vi "FPGA-SRAM-Top-Level.vi"() -> ()   [LabVIEW 2015]
uses:
  Typedefs/RadioData to SRAM states.ctl
  Typedefs/read from SRAM states.ctl
  <vilib>/Platform/TimedLoop/XDataNode/timing_clust.ctl
  <vilib>/Platform/TimedLoop/XDataNode/nitl_modes.ctl
  <vilib>/Platform/TimedLoop/XDataNode/wakeup.ctl
  <vilib>/rvi/Emulation/niFpgaSctlEmulationGetInTimedLoop.vi
  <vilib>/rvi/Emulation/niFpgaEmulationReportErrorSimple.vi
  <vilib>/rvi/Emulation/niFpgaGetClockAttributes.vi
  <vilib>/rvi/Emulation/niFpgaCriticalErrorInLSC.vi
  <vilib>/rvi/interface/RandomDataEmulation/niFpgaRandomDataHandleErrors.vi
  <vilib>/rvi/Emulation/niFpgaEmulationIsFPGAContextNoSignature.vi
  <vilib>/rvi/errors/niFpgaSetErrorForExecOnDevCompSimple.vi
  <vilib>/rvi/eio/common/nirviEmuReportErrorAndStop.vi
  <vilib>/rvi/DataTransferAndStorage/Container/Common/niFpgaContainerGetUniqueNameForEmu.vi
  <vilib>/rvi/FIFO/Fifo_Resource/nirvififoEmulationSetSize.vi
  <vilib>/rvi/FIFO/Fifo_Resource/nirviFifoEmulationQueueMgr.vi
  <instcachedir>/0/nirviFifoEmulationQueueMgr_E5CAEC123FF24DC58D834DCA3CDAA9B5.lvgen/nirviFifoEmulationQueueMgr_E5CAEC123FF24DC58D834DCA3CDAA9B5_001.vi
  <vilib>/rvi/FIFO/Fifo_Resource/nirvififoEmulationDetermineInputValidOut.vi
  <vilib>/rvi/FIFO/Fifo_Resource/nirvififoEmulationCreateLock.vi
  <vilib>/rvi/Emulation/niFpgaProcessEmulError.vi
  <vilib>/rvi/FIFO/Fifo_Resource/nirvififoEmulationObtainLock.vi
  <vilib>/rvi/FIFO/Fifo_Resource/nirvififoEmulationReleaseLock.vi
  <vilib>/rvi/occurrence/nirviWaitOnOccurrenceBase.vi
  <vilib>/rvi/errors/nirviReportUnexpectedCaseInternalError.vi
  <vilib>/rvi/errors/nirviReportUnexpectedCaseInternalError (U32).vi
  <vilib>/rvi/DataTransferAndStorage/Container/Common/niFpgaContainerSetEmuInfo.vi
  <vilib>/Utility/error.llb/Clear Errors.vi
  <vilib>/rvi/Memory/Memory_Emulation/nirvimemoryFastEmulation.vi
  <vilib>/rvi/Memory/Memory_Emulation/nirvimemoryEmulation.vi
  <vilib>/Platform/TimedLoop/XDataNode/XDataNode.xnode
  <vilib>/rvi/DataTransferAndStorage/Container/XNode/niFpgaContainer.xnode
  <vilib>/rvi/interface/RandomDataEmulation/nirviRandomDataFpgaReadWriteTemplate.vi
  <vilib>/rvi/FIFO/Fifo_Resource/nirvififoEmulationWrite.vi
  <vilib>/rvi/LocalResourceManager/LocalResourceManager.xnode
  <vilib>/rvi/FIFO/Fifo_Resource/nirvififoEmulationGetNumberOfElementsToRead.vi
  <vilib>/rvi/FIFO/Fifo_Resource/nirvififoEmulationRead.vi
  <vilib>/Platform/TimedLoop/XDataNode/XDNodeRunTimeDep.lvlib
  Shared/FPGA_shared.lvlib
  Typedefs/SRAM-typedefs.lvlib
  <instrlib>/_niInstr/Basic Elements/v1/FPGA/niInstr Basic Elements v1 FPGA.lvlib
panel:
  out "Target to Host Count":u32
  out "TH Timeout?":bool
  out "from SRAM timeout?":bool
  in  "Reset Read SRAM":bool=TRUE
  out "Radio Data Count to SRAM":u32
  out "Memory Write Address (indicator)":u32
  in  "Reset Write to SRAM":bool=TRUE
  out "HT Timeout?":bool
  out "Host to Target Count":u32
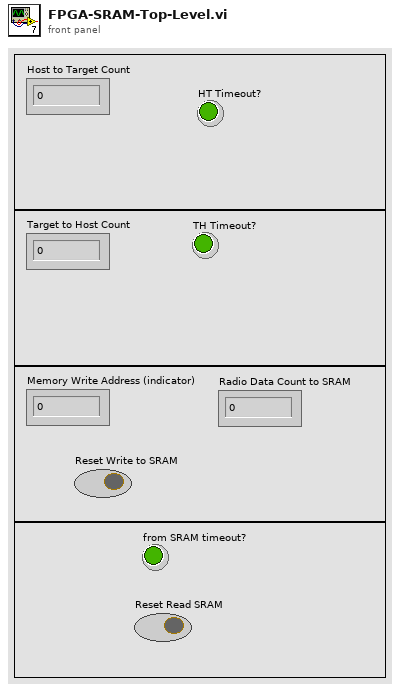
[diagram p1: front panel]
types:
  T1 = typedef "SRAM-typedefs.lvlib/read from SRAM states.ctl" = enum16{"idle", "read"}
  T2 = typedef "SRAM-typedefs.lvlib/RadioData to SRAM states.ctl" = enum16{"idle", "write", "reset"}
  T3 = typedef "XDNodeRunTimeDep.lvlib/timing_clust.ctl" = cluster{"Expected End [f-1]":u64, "Actual End [f-1]":u64, "Finished Late? [f-1]":bool, "Expected End [i-1]":u64, "Actual End [i-1]":u64, "Finished Late? [i-1]":bool, "Expected Start [i]":u64, "Actual Start [i]":u64, "Expected Start [f]":u64, "Actual Start [f]":u64, "Source Name":string, "Structure Name":string, "Period":i64, "Deadline":i64, "Offset":i64, "Start":i64, "Priority":i32, "Timeout":i32, "Mode":T4, "Wakeup Reason":T5, "Error":errorcluster, "Source Type":string, "Secondary Source Type":string, "Global End Time":u64, "Global Start Time":u64, "Frame Duration":u64, "Iteration Duration":u64, "Assigned CPU":i32, "I/O Scan Engine Mode":u32}
  T4 = typedef "XDNodeRunTimeDep.lvlib/nitl_modes.ctl" = enum32{"No Change", "Process missed periods, maintain original phase", "Discard missed periods, maintain original phase", "Process missed periods, ignore original phase", "Discard missed periods, ignore original phase"}
  T5 = typedef "XDNodeRunTimeDep.lvlib/wakeup.ctl" = enum32{"Normal", "Aborted", "Asynchronous wakeup", "Timing source error", "Timed loop error", "Timeout"}
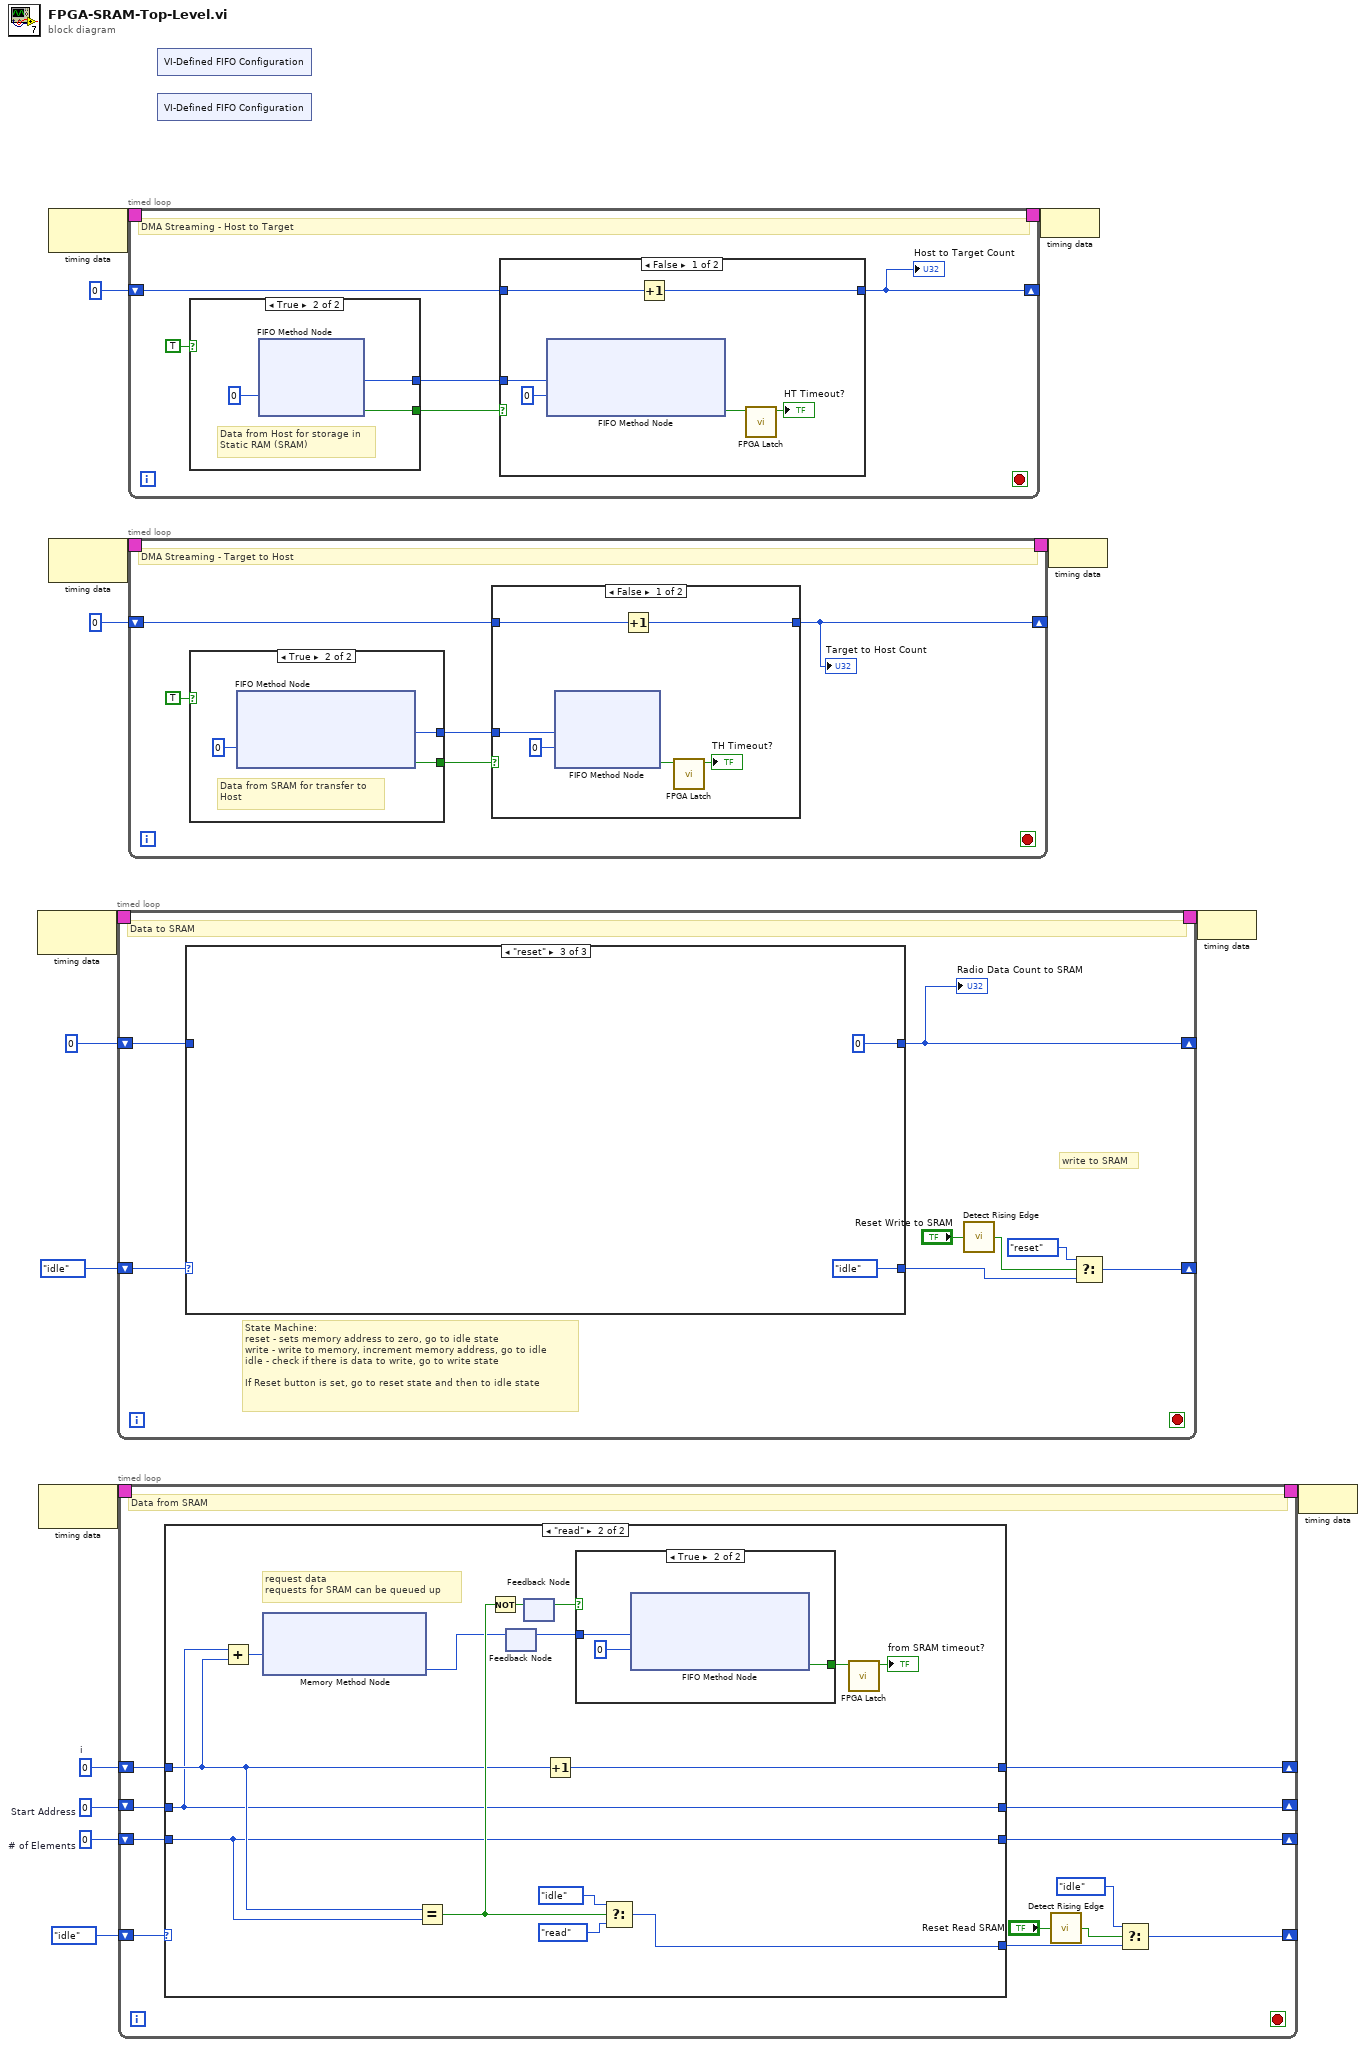
[diagram p0: block diagram]
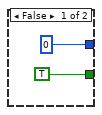
[diagram p2: hidden frame]
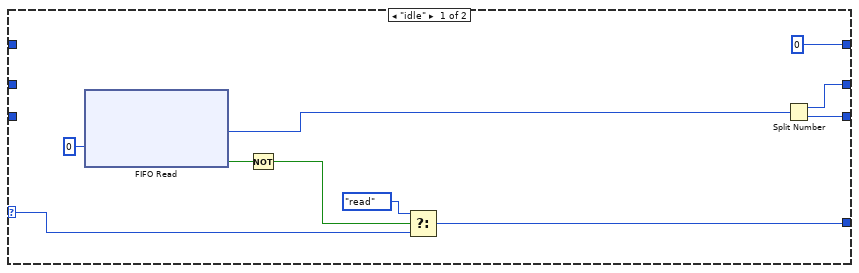
[diagram p4: hidden frame]
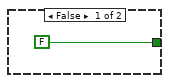
[diagram p5: hidden frame]
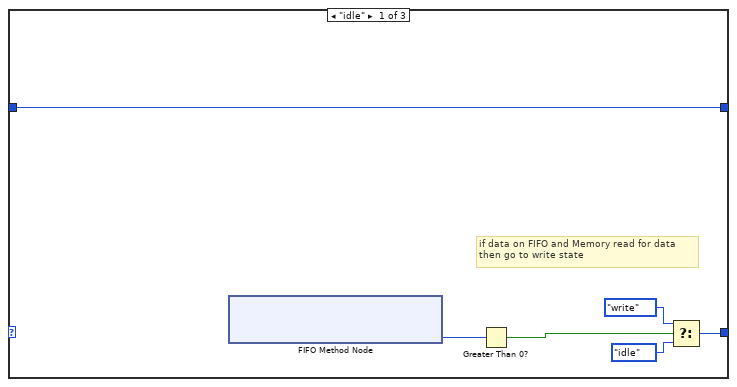
[diagram p6: hidden frame]
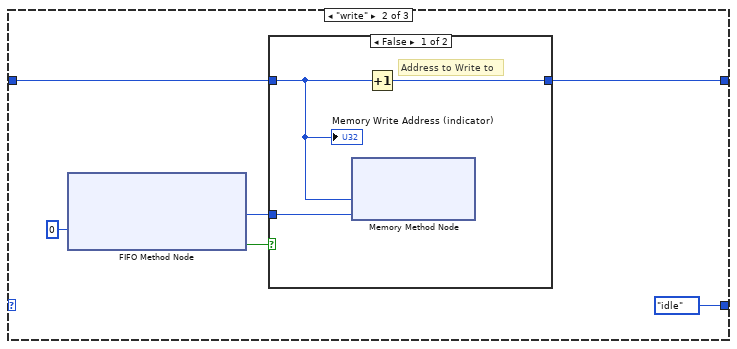
[diagram p7: hidden frame]
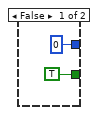
[diagram p9: hidden frame]
diagram:
  w1 = u32 0  # # of Elements
  w2 = u32 0  # Start Address
  w3 = u32 0  # i
  n1 = node-c288() -> (w13:T3)  [unwired: 1 in]
  n2 = node-c288() -> (w9:T3)  [unwired: 1 in]
  n3 = node-c288() -> (w16:T3)  [unwired: 1 in]
  n4 = node-c288() -> (w6:T3)  [unwired: 1 in]
  n5 = timed-loop {
    timing: w13 -> [_]
    timing-out: [_] -> w12
    shift-right: [w17] -> _
    shift-left: u32 0 ("Timeout") -> [w24]
    shift-right: [w19] -> _
    shift-left: RadioData_to_SRAM_states."idle" -> [w23]
    stop <- _ stop-if-true
    # "State Machine:\nreset - sets memory address to zero, go to idle state\nwrite - write to memory, increment memory address, go to idle\nidle - check if there is data to write, go to write state\n\nIf Reset button is set, go to reset state and then to idle state"
    # "write to SRAM"
    # "Data to SRAM"
    n6 = case shown="\"reset\"" w23 {
      tunnel: w24 -> [w30 w36 _]
      tunnel: [w30 w34 u32 0 ("Timeout")] -> w17
      tunnel: [w28 RadioData_to_SRAM_states."idle" RadioData_to_SRAM_states."idle"] -> w18
      frame "idle" {
        # "if data on FIFO and Memory read for data\nthen go to write state"
        n7 = xnode ("FIFO Method Node")() -> ("Number of Elements to Read"=w29:u32)  [unwired: 1 in, 1 out]
        n8 = Greater Than 0?(x=w29) -> (x > 0?=w25:bool)
        n9 = Select(t=RadioData_to_SRAM_states."write", s=w25, f=RadioData_to_SRAM_states."idle") -> (s? t:f=w28:T2)
      }
      frame "write" {
        n10 = xnode ("FIFO Method Node")("Timeout"=0) -> ("Element"=w31:u64, "Timed Out?"=w33:bool)  [unwired: 1 in, 1 out]
        n11 = case shown="False" w33 {
          tunnel: [w39 w40] -> w34
          tunnel: w36 -> [w38 w40]
          tunnel: w31 -> [w37 _]
          frame False {
            # "Address to Write to"
            n12 = xnode ("Memory Method Node")("Address"=w38, "Data"=w37) -> ()  [unwired: 2 in, 2 out]
            n13 = Increment(x=w38) -> (x+1=w39:u32)
            "Memory Write Address (indicator)" <- w38
          }
          frame True {
          }
        }
      }
      frame "reset" {
      }
    }
    "Radio Data Count to SRAM" <- w17
    n14 = call <instrlib>:"Detect Rising Edge.vi"("signal"="Reset Write to SRAM") -> ("edge detected"=w20:bool)  [unwired: 14 in]
    n15 = Select(t=RadioData_to_SRAM_states."reset", s=w20, f=w18) -> (s? t:f=w19:T2)
  }
  n16 = timed-loop {
    timing: w9 -> [_]
    timing-out: [_] -> w8
    shift-right: [w52] -> _
    shift-left: read_from_SRAM_states."idle" ("read from DRAM states") -> [w56]
    shift-right: [w47] -> _
    shift-left: w2 -> [w49]
    shift-right: [w45] -> _
    shift-left: w1 -> [w48]
    shift-right: [w46] -> _
    shift-left: w3 -> [w50]
    stop <- _ stop-if-true
    # "Data from SRAM"
    n17 = case shown="\"read\"" w56 {
      selector: w56 -> [w65 _]
      tunnel: [w66 w81] -> w53
      tunnel: w50 -> [_ w73]
      tunnel: w49 -> [_ w72]
      tunnel: w48 -> [_ w71]
      tunnel: [w58 w71] -> w45
      tunnel: [w59 w72] -> w47
      tunnel: [u32 0 w67] -> w46
      frame "idle" {
        n18 = xnode "FIFO Read"("Timeout"=0) -> ("Element"=w60:u64, "Timed Out?"=w62:bool)  [unwired: 1 in, 1 out]
        n19 = Not(x=w62) -> (.not. x?=w61:bool)
        n20 = Select(t=read_from_SRAM_states."read" ("read from DRAM states"), s=w61, f=w65) -> (s? t:f=w66:T1)
        n21 = Split Number(x=w60) -> (hi(x)=w59:u32, lo(x)=w58:u32)
      }
      frame "read" {
        # "request data\nrequests for SRAM can be queued up"
        n22 = Add(x=w72, y=w73) -> (x+y=w69:u32)
        n23 = xnode ("Memory Method Node")("Address"=w69) -> ("Data"=w68:u64)  [unwired: 1 in, 1 out]
        n24 = Equal?(x=w73, y=w71) -> (x = y?=w75:bool)
        n25 = Not(x=w75) -> (.not. x?=w74:bool)
        n26 = feedback-in #1(w68) -> ()
        n27 = feedback #1() -> (w76:u64)  [unwired: 1 in]
        n28 = feedback-in #2(w74) -> ()
        n29 = feedback #2() -> (w70:bool)  [unwired: 1 in]
        n30 = Increment(x=w73) -> (x+1=w67:u32)
        n31 = case shown="True" w70 {
          tunnel: [FALSE ("Timed Out?") w85] -> w77
          tunnel: w76 -> [_ w83]
          frame False {
          }
          frame True {
            n32 = xnode ("FIFO Method Node")("Element"=w83, "Timeout"=0) -> ("Timed Out?"=w85:bool)  [unwired: 1 in, 1 out]
          }
        }
        n33 = Select(t=read_from_SRAM_states."idle" ("read from DRAM states"), s=w75, f=read_from_SRAM_states."read" ("read from DRAM states")) -> (s? t:f=w81:T1)
        n34 = call "FPGA Latch.vi"("Input"=w77) -> ("Latch?"=→"from SRAM timeout?":bool)  [unwired: 10 in]
      }
    }
    n35 = call <instrlib>:"Detect Rising Edge.vi"("signal"="Reset Read SRAM") -> ("edge detected"=w54:bool)  [unwired: 14 in]
    n36 = Select(t=read_from_SRAM_states."idle" ("read from DRAM states"), s=w54, f=w53) -> (s? t:f=w52:T1)
  }
  n37 = timed-loop {
    timing: w16 -> [_]
    timing-out: [_] -> w15
    shift-right: [w91] -> _
    shift-left: u32 0 -> [w92]
    stop <- _ stop-if-true
    # "DMA Streaming - Host to Target"
    n38 = case shown="True" TRUE {
      tunnel: [u64 0 ("Element") w97] -> w89
      tunnel: [TRUE ("Timed Out?") w96] -> w90
      frame False {
      }
      frame True {
        # "Data from Host for storage in\nStatic RAM (SRAM)"
        n39 = xnode ("FIFO Method Node")("Timeout"=0) -> ("Element"=w97:u64, "Timed Out?"=w96:bool)  [unwired: 1 in, 1 out]
      }
    }
    n40 = case shown="False" w90 {
      tunnel: w89 -> [w99 _]
      tunnel: w92 -> [w103 w104]
      tunnel: [w98 w104] -> w91
      frame False {
        n41 = xnode ("FIFO Method Node")("Element"=w99, "Timeout"=0) -> ("Timed Out?"=w101:bool)  [unwired: 1 in, 1 out]
        n42 = Increment(x=w103) -> (x+1=w98:u32)
        n43 = call "FPGA Latch.vi"("Input"=w101) -> ("Latch?"=→"HT Timeout?":bool)  [unwired: 10 in]
      }
      frame True {
      }
    }
    "Host to Target Count" <- w91
  }
  n44 = timed-loop {
    timing: w6 -> [_]
    timing-out: [_] -> w5
    shift-right: [w107] -> _
    shift-left: u32 0 -> [w108]
    stop <- _ stop-if-true
    # "DMA Streaming - Target to Host"
    n45 = case shown="True" TRUE {
      tunnel: [u64 0 ("Element") w116] -> w110
      tunnel: [TRUE ("Timed Out?") w115] -> w111
      frame False {
      }
      frame True {
        # "Data from SRAM for transfer to\nHost"
        n46 = xnode ("FIFO Method Node")("Timeout"=0) -> ("Element"=w116:u64, "Timed Out?"=w115:bool)  [unwired: 1 in, 1 out]
      }
    }
    n47 = case shown="False" w111 {
      tunnel: w110 -> [w119 _]
      tunnel: w108 -> [w118 w123]
      tunnel: [w117 w123] -> w107
      frame False {
        n48 = xnode ("FIFO Method Node")("Element"=w119, "Timeout"=0) -> ("Timed Out?"=w121:bool)  [unwired: 1 in, 1 out]
        n49 = Increment(x=w118) -> (x+1=w117:u32)
        n50 = call "FPGA Latch.vi"("Input"=w121) -> ("Latch?"=→"TH Timeout?":bool)  [unwired: 10 in]
      }
      frame True {
      }
    }
    "Target to Host Count" <- w107
  }
  n51 = xnode "VI-Defined FIFO Configuration"() -> ()  [unwired: 1 out]
  n52 = xnode "VI-Defined FIFO Configuration"() -> ()  [unwired: 1 out]
  n53 = node-c288(w15) -> ()
  n54 = node-c288(w5) -> ()
  n55 = node-c288(w12) -> ()
  n56 = node-c288(w8) -> ()
